vi "Apply VNS to Best Solution.vi"(7 "Max Allowed Time Passed?":bool, 8 "error in (no error)":errorcluster, 9 "Scheduler.lvclass":refnum<class "Scheduler.lvclass">, 10 "GA in":refnum<class "GA.lvclass">, 11 "OSSP_Problem in":refnum<class "OSSP_Problem.lvclass">) -> (0 "error out":errorcluster, 1 "Scheduler.lvclass Out":refnum<class "Scheduler.lvclass">, 2 "GA out":refnum<class "GA.lvclass">, 3 "OSSP_Problem out":refnum<class "OSSP_Problem.lvclass">)   [LabVIEW 2013]
uses:
  Classes/OSSP_Problem.lvclass
  Classes/GA.lvclass
  Classes/Scheduler.lvclass
  Classes/GA.lvclass/GA.ctl
  Classes/Scheduler.lvclass/Scheduler.ctl
  Classes/OSSP_Problem.lvclass/OSSP_Problem.ctl
  Insert Neighborhood.vi
  Inversion Neighborhood.vi
  Zobolas Local Search Engine.vi
  Classes/OSSP_Problem_Class/Getters/Read Number of Machines.vi
  Global Schedule Selector.vi
  GA/SubVIS/Remove Duplicates In Array.vi
  Generate Two Indices for Local Search.vi
  Or-Opt(Zobolas) Neighborhood.vi
  Swap Neighborhood.vi
  Classes/Scheduler_Class/NonDelay Scheduler/Non Delay Scheduler Engine.vi
  Classes/OSSP_Problem_Class/Getters/Read Number of Jobs.vi
  Classes/OSSP_Problem_Class/Getters/Read Processing Times.vi
  GA/SubVIS/Calcualte General Tardiness.vi
  Classes/OSSP_Problem_Class/Getters/Read Due Dates.vi
  Classes/Scheduler_Class/Giffler Thompson Active Schedule Engine.vi
  Classes/Scheduler_Class/Prins FIFO Scheduler Methods and Controls/Methods/Calculate Makespan (Prins FIFO Engine).vi
  Classes/Scheduler_Class/Prins FIFO Scheduler Methods and Controls/Methods/Calculate Tardiness (Prins FIFO Engine).vi
  Classes/Scheduler_Class/Modified GT Active Scheduler/GT Active Scheduler wSubset4Tardiness.vi
  Classes/Scheduler_Class/Getters/Read Lambda.vi
  Classes/Scheduler_Class/Getters/Read Operation Selection Rule.vi
  Classes/Scheduler_Class/Getters/Read Scheduler.vi
  Classes/Scheduler_Class/Operation to Machine Job Tuple.vi
  Classes/Scheduler_Class/Prins FIFO Scheduler Methods and Controls/Prins FIFO Scheduler.vi
  Classes/Scheduler_Class/Prins FIFO Scheduler Methods and Controls/Methods/Calculate Final Completion Times of Jobs.vi
  Classes/Scheduler_Class/Prins FIFO Scheduler Methods and Controls/Methods/Reorder Schedule(Prins FIFO) based on Start Times.vi
  Classes/Scheduler_Class/Modified GT Active Scheduler/GT Find Subset of Operations.vi
  Classes/Scheduler_Class/Modified GT Active Scheduler/Select Operation to Schedule Based on Rule.vi
  Classes/Scheduler_Class/Prins FIFO Scheduler Methods and Controls/Methods/UpdateMachineGaps.vi
  Classes/Scheduler_Class/Prins FIFO Scheduler Methods and Controls/Methods/UpdateJobGaps.vi
  Classes/Scheduler_Class/Prins FIFO Scheduler Methods and Controls/Methods/Find Intersecting Gaps.vi
  Classes/Scheduler_Class/GT Algorithm Find M_ok and J_ok.vi
  Classes/Scheduler_Class/Prins FIFO Scheduler Methods and Controls/Methods/Transform to Plain Job and Machine Gaps Array.vi
  Classes/Scheduler_Class/Semiactive Scheduler/Semi Active Scheduler Engine.vi
  Nonredundant Swap Neighborhood.vi
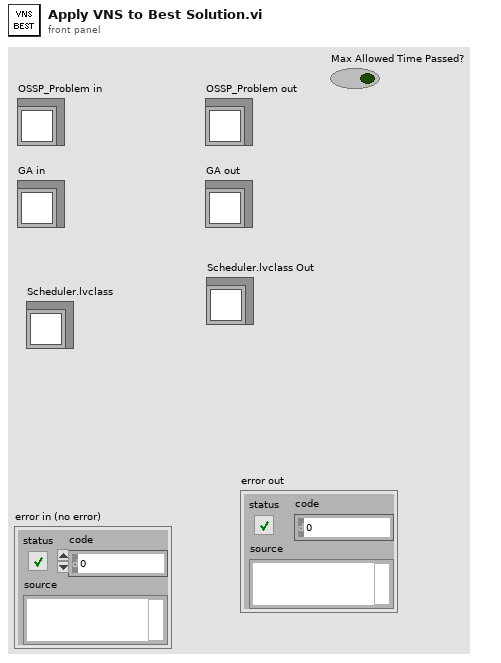
[diagram p1: front panel]
types:
  T1 = typedef "Solution_GA.ctl" = cluster{"Schedule":u16[], "Fitness":u16, "Fitness Valid?":bool}
  T2 = typedef "Objective.ctl" = enum16{"Makespan", "Total Tardiness"}
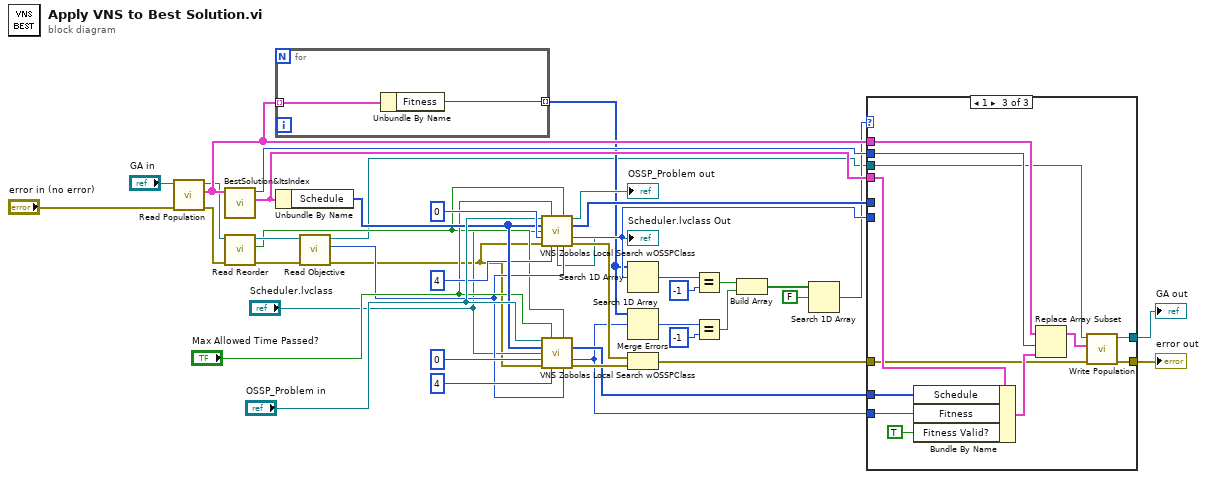
[diagram p0: block diagram]
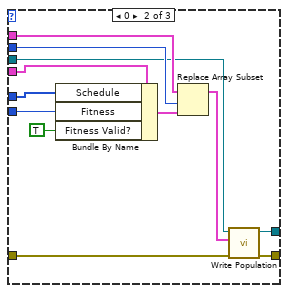
[diagram p3: hidden frame]
diagram:
  n1 = call "Read Population.vi"("error in (no error)"="error in (no error)", "GA in"="GA in") -> ("error out"=w28:errorcluster, "Population"=w34:T1[], "GA out"=w29:refnum<class "GA.lvclass">)  [unwired: 7 in]
  n2 = call "BestSolution&ItsIndex.vi"("Population"=w34) -> ("Best Solution In the Population"=w36:T1, "Best Solution Index for Replace"=w37:i32)  [unwired: 9 in]
  n3 = call "Read Reorder.vi"("error in (no error)"=w28, "GA in"=w29) -> ("error out"=w11:errorcluster, "Reorder"=w5:bool, "GA out"=w10:refnum<class "GA.lvclass">)  [unwired: 7 in]
  n4 = for {
    tunnel: w34 -> [w44] mode=indexing
    tunnel: [w43] -> w12 mode=indexing
    n5 = Unbundle By Name(w44) -> ("Fitness"=w43:u16)
  }
  n6 = Unbundle By Name(w36) -> ("Schedule"=w13:u16[])
  n7 = call "Read Objective .vi"("error in (no error)"=w11, "GA in"=w10) -> ("error out"=w3:errorcluster, "Objective"=w6:T2, "GA out"=w2:refnum<class "GA.lvclass">)  [unwired: 7 in]
  n8 = call "VNS Zobolas Local Search wOSSPClass.vi"("OSSP_Problem.lvclass"="OSSP_Problem in", "Max Allowed Time Passed?"="Max Allowed Time Passed?", "Reorder?"=w5, "Schedule In"=w13, "Scheduler.lvclass"="Scheduler.lvclass", "Max Iteration Count"=0, "error in (no error)"=w3, "Number of Neighborhoods"=4, "Objective"=w6) -> ("OSSP_Problem out"=→"OSSP_Problem out":refnum<class "OSSP_Problem.lvclass">, "VNS Result Out"=w35:u16[], "Makespan/Tardiness(FIFO Engine)"=w31:u16, "Scheduler.lvclass Out"=→"Scheduler.lvclass Out":refnum<class "Scheduler.lvclass">, "error out"=w27:errorcluster)  [unwired: 2 in]
  n9 = call "VNS Zobolas Local Search wOSSPClass.vi"("OSSP_Problem.lvclass"="OSSP_Problem in", "Max Allowed Time Passed?"="Max Allowed Time Passed?", "Reorder?"=w5, "Schedule In"=w13, "Scheduler.lvclass"="Scheduler.lvclass", "Max Iteration Count"=0, "error in (no error)"=w3, "Number of Neighborhoods"=4, "Objective"=w6) -> ("VNS Result Out"=w16:u16[], "Makespan/Tardiness(FIFO Engine)"=w15:u16, "error out"=w26:errorcluster)  [unwired: 2 in, 2 out]
  n10 = Search 1D Array(1D array=w12, element=w31) -> (index of element=w33:i32)  [unwired: 1 in]
  n11 = Search 1D Array(1D array=w12, element=w15) -> (index of element=w23:i32)  [unwired: 1 in]
  n12 = Merge Errors(w27, w26) -> (w25:errorcluster)
  n13 = Equal?(x=w33, y=-1) -> (x = y?=w21:bool)
  n14 = Equal?(x=w23, y=-1) -> (x = y?=w20:bool)
  n15 = Build Array(w21, w20) -> (w19:bool[])
  n16 = Search 1D Array(1D array=w19, element=FALSE) -> (index of element=w17:i32)  [unwired: 1 in]
  n17 = case shown="1" w17 {
    tunnel: w37 -> [_ w58 w70]
    tunnel: w36 -> [_ w57 w69]
    tunnel: w35 -> [_ w56 _]
    tunnel: w34 -> [_ w53 w66]
    tunnel: w25 -> [w45 w52 w65]
    tunnel: [w45 w51 w64] -> w41
    tunnel: w2 -> [w46 w49 w62]
    tunnel: [w46 w48 w61] -> w42
    tunnel: w31 -> [_ w47 _]
    tunnel: w16 -> [_ _ w60]
    tunnel: w15 -> [_ _ w59]
    frame -1, Default {
    }
    frame 0 {
      n18 = Bundle By Name(cluster=w57, "Schedule"=w56, "Fitness"=w47, "Fitness Valid?"=TRUE) -> (w54:T1)
      n19 = Replace Array Subset(array=w53, new element=w54, index=w58) -> (w50:T1[])
      n20 = call "Write Population.vi"("error in (no error)"=w52, "Population"=w50, "GA in"=w49) -> ("error out"=w51:errorcluster, "GA out"=w48:refnum<class "GA.lvclass">)  [unwired: 7 in]
    }
    frame 1 {
      n21 = Bundle By Name(cluster=w69, "Schedule"=w60, "Fitness"=w59, "Fitness Valid?"=TRUE) -> (w67:T1)
      n22 = Replace Array Subset(array=w66, new element=w67, index=w70) -> (w63:T1[])
      n23 = call "Write Population.vi"("error in (no error)"=w65, "Population"=w63, "GA in"=w62) -> ("error out"=w64:errorcluster, "GA out"=w61:refnum<class "GA.lvclass">)  [unwired: 7 in]
    }
  }
  "GA out" <- w42
  "error out" <- w41
